vi "Datasheet Calc Stat.vi"(11 "Channel Data":dbl[](array[numeric])) -> (0 "Maximum":dbl, 1 "Variance":dbl, 2 "Standard Deviation":dbl, 3 "Mean":dbl, 4 "Minimum":dbl, 5 "Median":dbl, 6 "N":dbl)   [LabVIEW 2011]
uses:
  <vilib>/Analysis/NI_AALBase.lvlib
panel:
  # "DELAY format data must be calculated prior to passing to this VI"
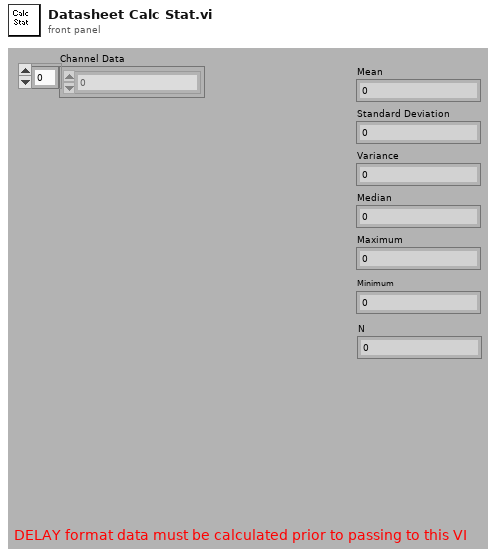
[diagram p1: front panel]
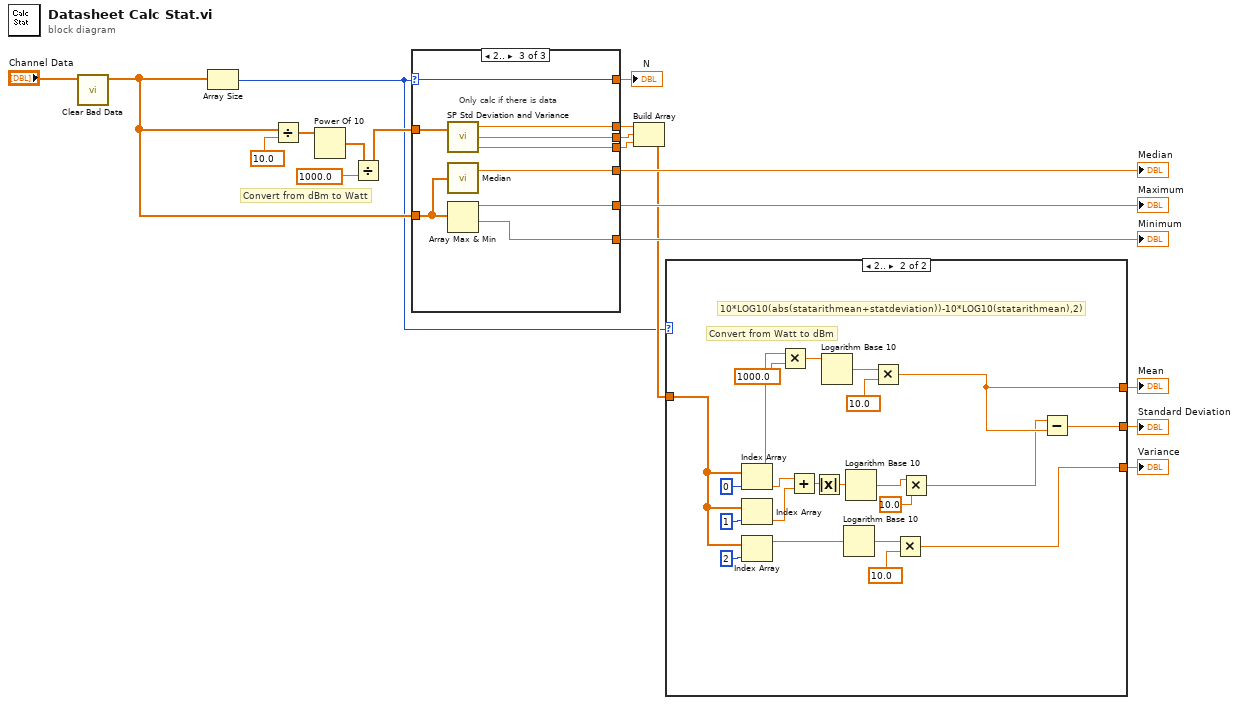
[diagram p0: block diagram]
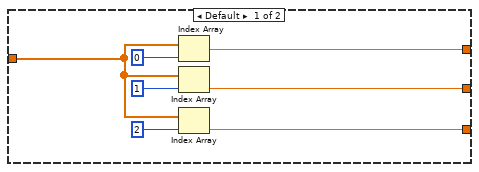
[diagram p2: hidden frame]
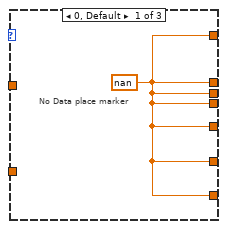
[diagram p3: hidden frame]
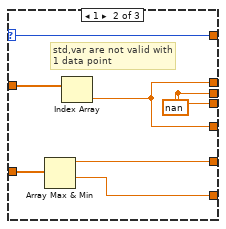
[diagram p4: hidden frame]
diagram:
  # "Convert from dBm to Watt"
  n1 = call "Clear Bad Data.vi"("Waveform IN"="Channel Data") -> ("Waveform out"=w16:dbl[])  [unwired: 10 out]
  n2 = Array Size(array=w16) -> (size(s)=w6:i32)
  n3 = Divide(x=w16, y=10.0) -> (x/y=w1:dbl[])
  n4 = Power Of 10(x=w1) -> (10^x=w2:dbl[])
  n5 = Divide(x=w2, y=1000.0) -> (x/y=w7:dbl[])
  n6 = case shown="2.." w6 {
    selector: w6 -> [_ w22 w28]
    tunnel: [w20 w23 w36] -> w19
    tunnel: [w20 w21 w35] -> w18
    tunnel: [w20 w21 w34] -> w17
    tunnel: [w20 w23 w33] -> w15
    tunnel: [w20 w27 w32] -> w14
    tunnel: [w20 w26 w31] -> w13
    tunnel: w16 -> [_ w25 w29]
    tunnel: w7 -> [_ w24 w30]
    tunnel: [w20 w22 w28] -> w5
    frame 0, Default {
      w20 = nan
      # "No Data place marker"
    }
    frame 1 {
      w21 = nan
      # "std,var are not valid with\n1 data point"
      n7 = Array Max & Min(array=w25) -> (max value=w27:dbl, min value=w26:dbl)  [unwired: 2 out]
      n8 = Index Array(array=w24) -> (element=w23:dbl)  [unwired: 1 in]
    }
    frame 2.. {
      # "Only calc if there is data"
      n9 = call "SP Std Deviation and Variance.vi"("X"=w30) -> ("mean"=w36:dbl, "standard deviation"=w35:dbl, "variance"=w34:dbl)  [unwired: 1 in]
      n10 = call <vilib>:"Median.vi"("X"=w29) -> ("median"=w33:dbl)  [unwired: 1 out]
      n11 = Array Max & Min(array=w29) -> (max value=w32:dbl, min value=w31:dbl)  [unwired: 2 out]
    }
  }
  "Minimum" <- w13
  "Maximum" <- w14
  "Median" <- w15
  "N" <- w5
  n12 = Build Array(w19, w18, w17) -> (w11:dbl[])
  n13 = case shown="2.." w6 {
    tunnel: w11 -> [w40 w64]
    tunnel: [w39 w63] -> w10
    tunnel: [w37 w62] -> w9
    tunnel: [w38 w61] -> w8
    frame Default {
      n14 = Index Array(array=w40, index=0) -> (element=w39:dbl)
      n15 = Index Array(array=w40, index=1) -> (element=w38:dbl)
      n16 = Index Array(array=w40, index=2) -> (element=w37:dbl)
    }
    frame 2.. {
      # "10*LOG10(abs(statarithmean+statdeviation))-10*LOG10(statarithmean),2)"
      # "Convert from Watt to dBm"
      n17 = Index Array(array=w64, index=0) -> (element=w44:dbl)
      n18 = Index Array(array=w64, index=1) -> (element=w54:dbl)
      n19 = Index Array(array=w64, index=2) -> (element=w45:dbl)
      n20 = Multiply(x=w44, y=1000.0) -> (x*y=w59:dbl)
      n21 = Add(x=w44, y=w54) -> (x+y=w51:dbl)
      n22 = Absolute Value(x=w51) -> (abs(x)=w50:dbl)
      n23 = Logarithm Base 10(1:w59) -> (0:w57:dbl)
      n24 = Logarithm Base 10(1:w45) -> (0:w47:dbl)
      n25 = Logarithm Base 10(1:w50) -> (0:w53:dbl)
      n26 = Multiply(x=w57, y=10.0) -> (x*y=w63:dbl)
      n27 = Multiply(x=w47, y=10.0) -> (x*y=w62:dbl)
      n28 = Multiply(x=w53, y=10.0 ("index")) -> (x*y=w49:dbl)
      n29 = Subtract(x=w49, y=w63) -> (x-y=w61:dbl)
    }
  }
  "Variance" <- w9
  "Standard Deviation" <- w8
  "Mean" <- w10
